vi "Load LVTest File.vi"(8 "error in (no error)":errorcluster, 10 "LVTest file":path, 11 "LUnit Test Vector In":refnum<class "LUnit Test Vector.lvclass">) -> (0 "error out":errorcluster, 1 "Test Case Table":string[][](array[string]), 2 "File Contents":string[][](array[string]), 3 "LUnit Test Vector Out":refnum<class "LUnit Test Vector.lvclass">)   [LabVIEW 2020, in "LUnit Test Vector.lvclass"]
uses:
  LUnit Test Vector.lvclass
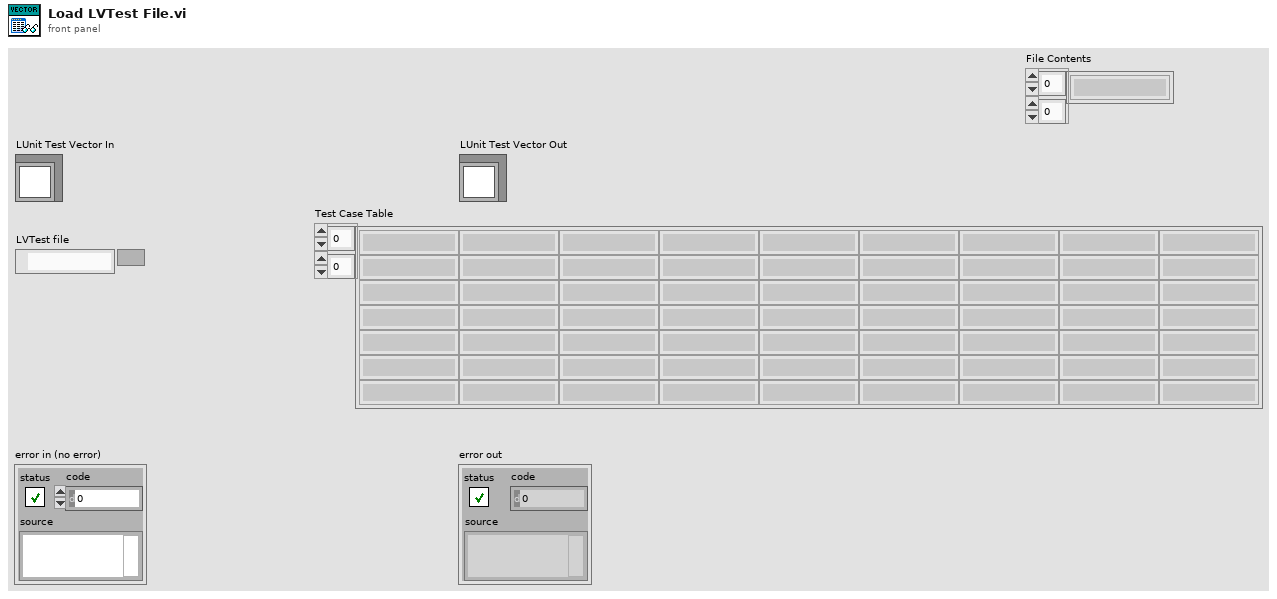
[diagram p1: front panel]
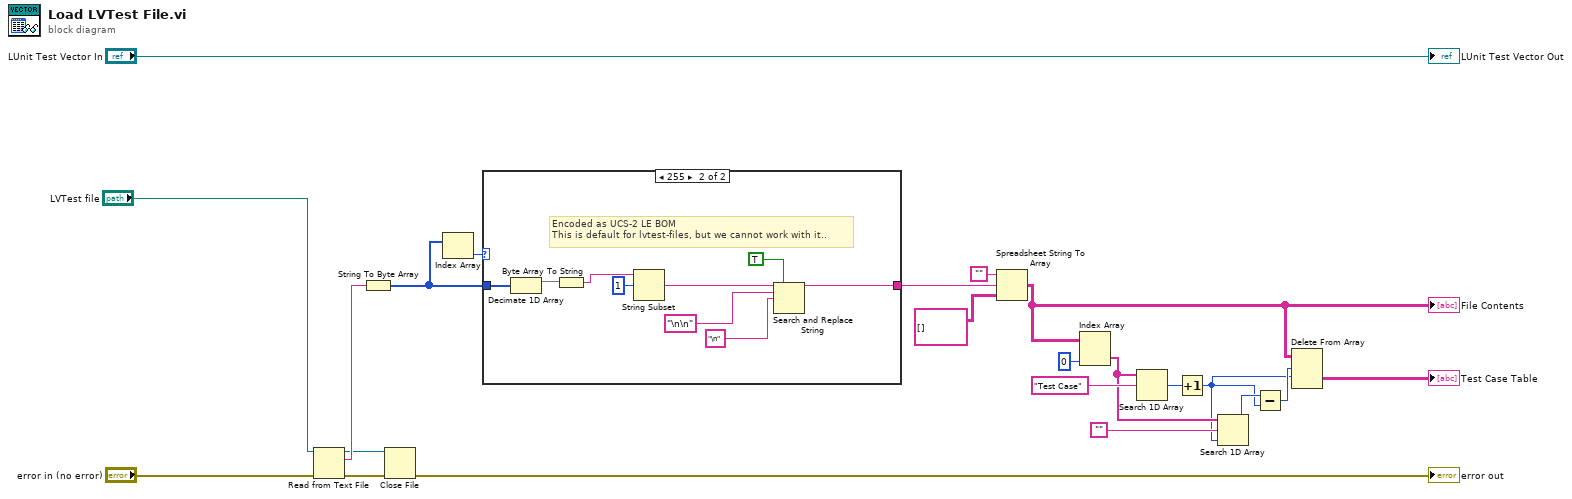
[diagram p0: block diagram]
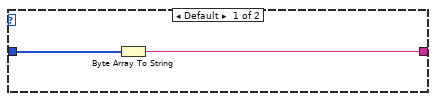
[diagram p2: hidden frame]
diagram:
  n1 = Read from Text File(file (use dialog)="LVTest file", error in="error in (no error)") -> (refnum out=w17:refnum<file>, text=w20:string, error out=w16:errorcluster)  [unwired: 2 in, 1 out]
  n2 = String To Byte Array(string=w20) -> (unsigned byte array=w19:u8[])
  n3 = Close File(refnum=w17, error in=w16) -> (error out=→"error out":errorcluster)  [unwired: 1 out]
  n4 = Index Array(array=w19) -> (element=w18:u8)  [unwired: 1 in]
  n5 = case shown="255" w18 {
    tunnel: [w23 w28] -> w12
    tunnel: w19 -> [w24 w30]
    frame Default {
      n6 = Byte Array To String(unsigned byte array=w24) -> (string=w23:string)
    }
    frame 255 {
      # "Encoded as UCS-2 LE BOM\nThis is default for lvtest-files, but we cannot work with it.."
      n7 = Decimate 1D Array(w30) -> (w33:u8[])  [unwired: 1 out]
      n8 = Byte Array To String(unsigned byte array=w33) -> (string=w31:string)
      n9 = String Subset(string=w31, offset (0)=1) -> (substring=w29:string)  [unwired: 1 in]
      n10 = Search and Replace String(replace all?=TRUE ("replace all? (F)"), input string=w29, search string="\n\n", replace string="\n" ("search string")) -> (result string=w28:string)  [unwired: 4 in, 3 out]
    }
  }
  n11 = Spreadsheet String To Array(format string="", spreadsheet string=w12, array type (2D Dbl)=string[][] []) -> (array=w3:string[][])  [unwired: 1 in]
  "File Contents" <- w3
  n12 = Index Array(array=w3, index (col)=0 ("disabled index (col)")) -> (element=w7:string[])  [unwired: 1 in]
  n13 = Search 1D Array(1D array=w7, element="Test Case") -> (index of element=w5:i32)  [unwired: 1 in]
  n14 = Increment(x=w5) -> (x+1=w1:i32)
  n15 = Search 1D Array(1D array=w7, element="", start index (0)=w1) -> (index of element=w6:i32)
  n16 = Subtract(x=w6, y=w1) -> (x-y=w4:i32)
  n17 = Delete From Array(array=w3, length=w4, index (row)=w1) -> (deleted portion=→"Test Case Table":string[][])  [unwired: 1 in, 1 out]
  "LUnit Test Vector Out" <- "LUnit Test Vector In"
